vi "Read Alert Values.vi"(1 "Section":i32) -> (0 "Temp Warning Values":T1)   [LabVIEW 2017, in "GUI.lvlib"]
uses:
  GUI.lvlib
  <vilib>/Utility/config.llb/NI_LVConfig.lvlib
panel:
  in  "TxO":T2
  in  "TxA":T3
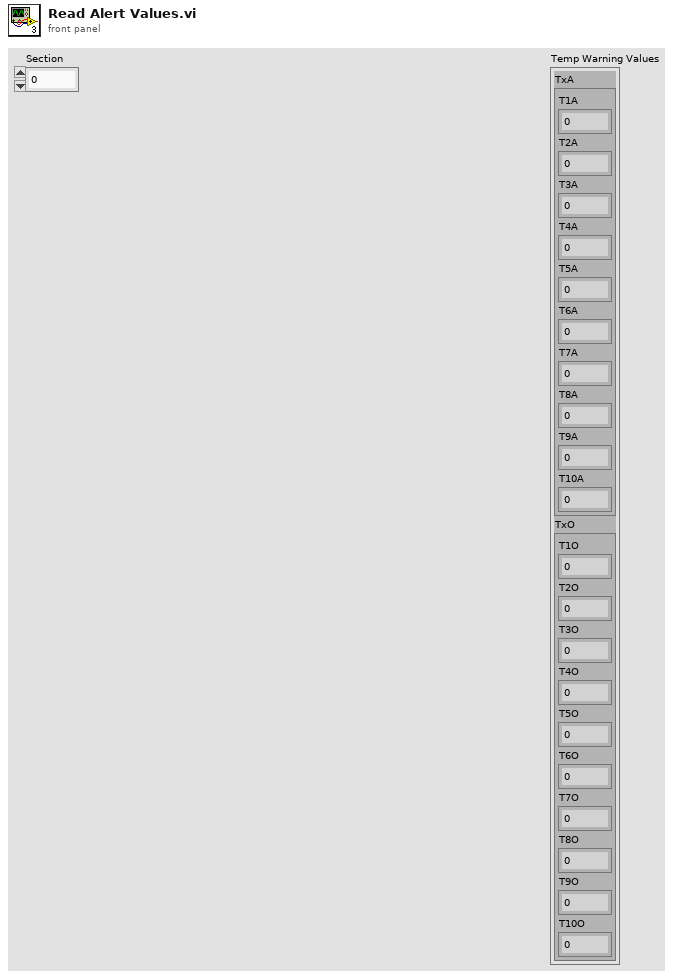
[diagram p1: front panel]
types:
  T1 = cluster{"TxA":cluster{"T1A":dbl, "T2A":dbl, "T3A":dbl, "T4A":dbl, "T5A":dbl, "T6A":dbl, "T7A":dbl, "T8A":dbl, "T9A":dbl, "T10A":dbl}, "TxO":cluster{"T1O":dbl, "T2O":dbl, "T3O":dbl, "T4O":dbl, "T5O":dbl, "T6O":dbl, "T7O":dbl, "T8O":dbl, "T9O":dbl, "T10O":dbl}}
  T2 = cluster{"T1O":dbl, "T2O":dbl, "T3O":dbl, "T4O":dbl, "T5O":dbl, "T6O":dbl, "T7O":dbl, "T8O":dbl, "T9O":dbl, "T10O":dbl}
  T3 = cluster{"T1A":dbl, "T2A":dbl, "T3A":dbl, "T4A":dbl, "T5A":dbl, "T6A":dbl, "T7A":dbl, "T8A":dbl, "T9A":dbl, "T10A":dbl}
  T4 = typedef "NI_LVConfig.lvlib/Config Data RefNum.ctl" = refnum<k1>
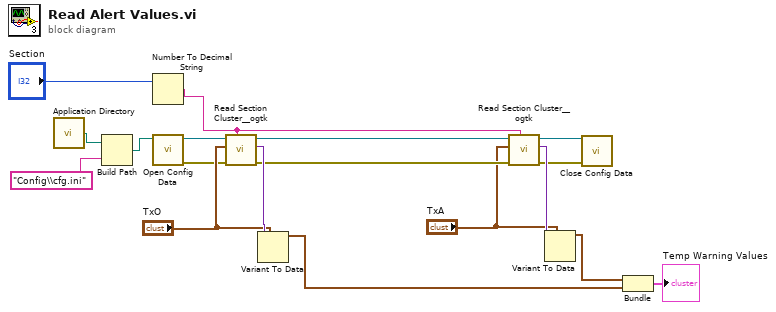
[diagram p0: block diagram]
diagram:
  n1 = call <vilib>:"Application Directory.vi"() -> ("Application Directory"=w16:path)
  n2 = Build Path(base path=w16, name or relative path="Config\\cfg.ini") -> (appended path=w14:path)
  n3 = Number To Decimal String(number="Section") -> (decimal integer string=w9:string)  [unwired: 1 in]
  n4 = call <vilib>:"Open Config Data.vi"("configuration file path"=w14) -> ("error out"=w3:errorcluster, "refnum"=w2:T4)  [unwired: 8 in, 1 out]
  n5 = call <userlib>:"Read Section Cluster__ogtk.vi"("section (optional)"=w9, "error in (no error)"=w3, "Section Formatted Cluster Type"="TxO", "refnum"=w2) -> ("error out"=w10:errorcluster, "Section Formatted Cluster"=w12:variant, "dup refnum"=w13:T4)  [unwired: 3 in, 2 out]
  n6 = Variant To Data(type="TxO", Variant=w12) -> (data=w17:T2)  [unwired: 1 in, 1 out]
  n7 = call <userlib>:"Read Section Cluster__ogtk.vi"("section (optional)"=w9, "error in (no error)"=w10, "Section Formatted Cluster Type"="TxA", "refnum"=w13) -> ("error out"=w5:errorcluster, "Section Formatted Cluster"=w11:variant, "dup refnum"=w4:T4)  [unwired: 3 in, 2 out]
  n8 = Variant To Data(type="TxA", Variant=w11) -> (data=w18:T3)  [unwired: 1 in, 1 out]
  n9 = call <vilib>:"Close Config Data.vi"("error in (no error)"=w5, "refnum"=w4) -> ()  [unwired: 8 in, 2 out]
  n10 = Bundle("TxA"=w18, "TxO"=w17) -> (→"Temp Warning Values":T1)  [unwired: 1 in]
